vi "EXAMPLE APPLICATION.vi"() -> ()   [LabVIEW 2021]
uses:
  <vilib>/Instr/_visa.llb/VISA Configure Serial Port (Instr).vi
panel:
  out "(hi.lo)":u16
  out "Potentiometer:":dbl(knob) scale=0.0..1023.0
  in  "Start":bool
  in  "Write Test:":i32[](array[numeric])
  in  "Write?":bool
  out "DBarray":dbl[][](array[numeric])
  in  "DB File":string="cansart_db.h"
  in  "stop":bool
  in  "BaudRate:":u32=115200
  in  "COM:":refnum<visa-resource-name>
  # "Cansart Example Application"
  # "Test Potentiometer by connecting a potentiometer\non the pin referred on your controller example"
  # "Double Click on the 1023 number to change it \nto a higher number depending on what your \nADC resolution"
  # "Engineered and Maintained by:\nGuilherme Candido\nteoriaeletrica@gmail.com"
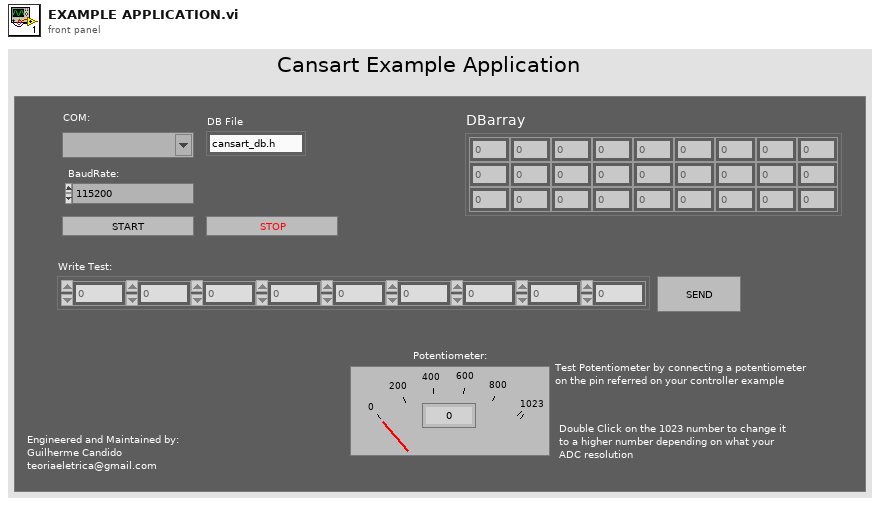
[diagram p1: front panel]
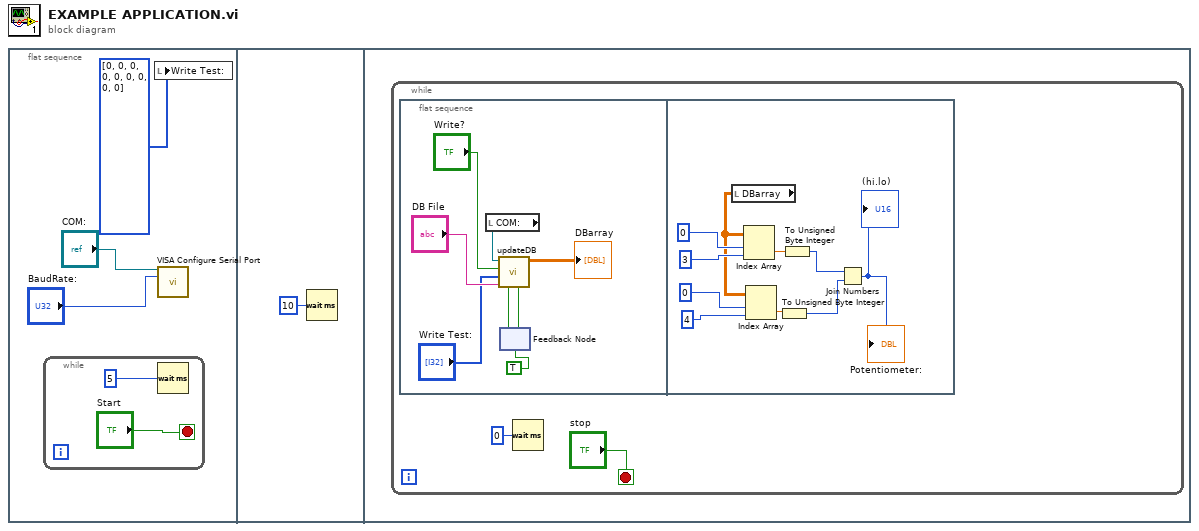
[diagram p0: block diagram]
diagram:
  n1 = flat-sequence {
    frame #0 {
      n2 = while {
        stop <- "Start" stop-if-true
        n3 = Wait (ms)(milliseconds to wait=u32 5) -> ()  [unwired: 1 out]
      }
      n4 = local write "Write Test:"(i32[] [0, 0, 0, 0, 0, 0, 0, 0, 0] ("Data Write")) -> ()
      n5 = call-poly "VISA Configure Serial Port"("VISA resource name"="COM:", "baud rate (9600)"="BaudRate:") -> ()  [unwired: 12 in, 2 out]
    }
    frame #1 {
      n6 = Wait (ms)(milliseconds to wait=u32 10) -> ()  [unwired: 1 out]
    }
    frame #2 {
      n7 = while {
        stop <- "stop" stop-if-true
        n8 = flat-sequence {
          frame #0 {
            n9 = local read "COM:"() -> (w16:refnum<visa-resource-name>)
            n10 = feedback #1(TRUE ("First 2")) -> (w10:bool)
            n11 = call "updateDB.vi"("First"=w10, "DBname"="DB File", "Data Write"="Write Test:", "Write?"="Write?", "COM PORT"=w16) -> ("DBarray"=→"DBarray":dbl[][], "First 2"=w11:bool)  [unwired: 5 in]
            n12 = feedback-in #1(w11) -> ()
          }
          frame #1 {
            n13 = local read "DBarray"() -> (w24:dbl[][])
            n14 = Index Array(array=w24, index (row)=0, index (col)=3 ("disabled index (col)")) -> (element=w21:dbl)
            n15 = Index Array(array=w24, index (row)=0, index (col)=4 ("disabled index (col)")) -> (element=w19:dbl)
            n16 = To Unsigned Byte Integer(number=w19) -> (unsigned 8bit integer=w18:u8)
            n17 = To Unsigned Byte Integer(number=w21) -> (unsigned 8bit integer=w20:u8)
            n18 = Join Numbers(hi=w20, lo=w18) -> ((hi.lo)=→"(hi.lo)" →"Potentiometer:":u16)
          }
        }
        n19 = Wait (ms)(milliseconds to wait=u32 0) -> ()  [unwired: 1 out]
      }
    }
  }
